vi "sinh fitter.vi"(3 "iterations":u16=1 min=1, 4 "1/B":dbl format="%.3f", 5 "amp.":dbl[](array[numeric]) format="%.2f", 6 "T":dbl[](array[numeric]) format="%.2f") -> (0 "sum of square deviations":dbl format="%.2f", 1 "a":dbl format="%.2f", 2 "m*":dbl format="%.2f")   [LabVIEW 2016]
uses:
  <vilib>/Analysis/baseanly.llb/Real Dot Product.vi
  <vilib>/Analysis/NI_AALBase.lvlib
  <vilib>/Analysis/NI_AALPro.lvlib
panel:
  out "plotted data":cluster{dbl[], dbl[]}[](graph)
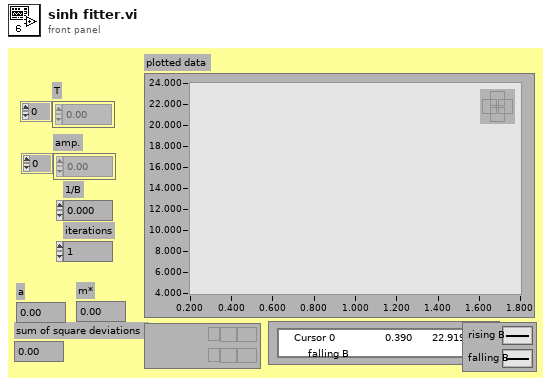
[diagram p1: front panel]
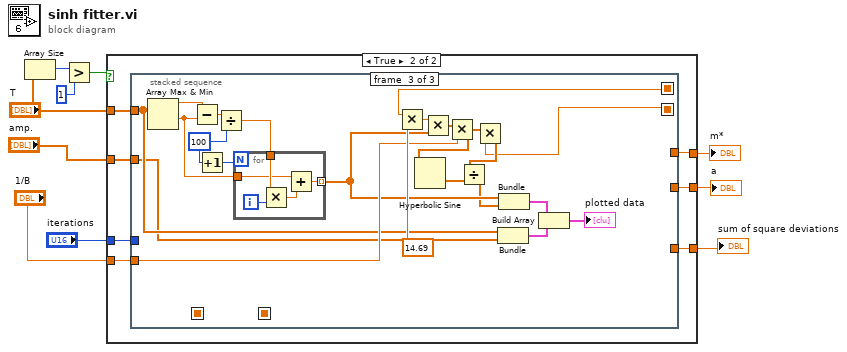
[diagram p0: block diagram]
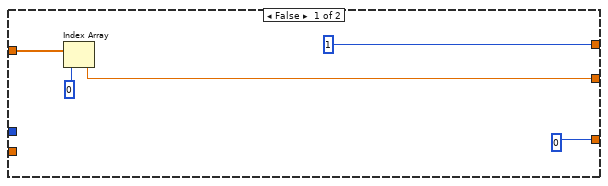
[diagram p2: hidden frame]
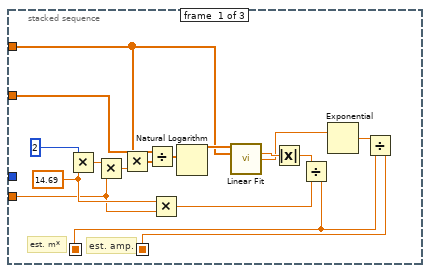
[diagram p3: hidden frame]
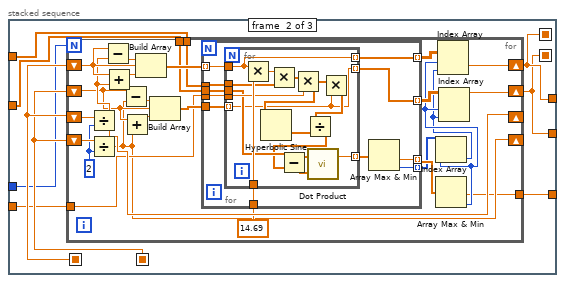
[diagram p4: hidden frame]
diagram:
  n1 = Array Size(array="T") -> (size(s)=w8:i32)
  n2 = Greater?(x=w8, y=1) -> (0:w7:bool)
  n3 = case shown="True" w7 {
    tunnel: [1 w19] -> w6
    tunnel: "T" -> [_ w22]
    tunnel: "amp." -> [w13 w21]
    tunnel: "1/B" -> [_ w20]
    tunnel: "iterations" -> [_ w18]
    tunnel: [w12 w17] -> w2
    tunnel: [0 w16] -> w1
    frame False {
      n4 = Index Array(array=w13, index=0) -> (element=w12:dbl)
    }
    frame True {
      n5 = stacked-sequence {
        seq-local: [w23 _ _] -> [_ w48 _]
        seq-local: [w24 _ _] -> [_ w47 _]
        seq-local: [_ w41 _] -> [_ _ w109]
        seq-local: [_ w40 _] -> [_ _ w107]
        tunnel: w22 -> [w32 w46 w104]
        tunnel: w21 -> [w35 w44 w103]
        tunnel: w20 -> [w30 w45 w108]
        tunnel: [_ w41 _] -> w19
        tunnel: w18 -> [_ w43 _]
        tunnel: [_ w40 _] -> w17
        tunnel: [_ w42 _] -> w16
        frame #0 {
          w31 = 14.69
          # "est. amp."
          # "est. m*"
          n6 = Multiply(x=2, y=w31) -> (x*y=w38:dbl)
          n7 = Multiply(x=w38, y=w30) -> (x*y=w37:dbl)
          n8 = Multiply(x=w32, y=w37) -> (x*y=w36:dbl[])
          n9 = Divide(x=w35, y=w36) -> (x/y=w34:dbl[])
          n10 = Multiply(x=w31, y=w30) -> (x*y=w28:dbl)
          n11 = Natural Logarithm(1:w34) -> (0:w33:dbl[])
          n12 = call <vilib>:"Linear Fit.vi"("Y"=w33, "X"=w32) -> ("slope"=w29:dbl, "intercept"=w26:dbl)  [unwired: 9 in, 3 out]
          n13 = Absolute Value(x=w29) -> (abs(x)=w27:dbl)
          n14 = Divide(x=w27, y=w28) -> (x/y=w23:dbl)
          n15 = Exponential(1:w26) -> (0:w25:dbl)
          n16 = Divide(x=w25, y=w23) -> (x/y=w24:dbl)
        }
        frame #1 {
          n17 = for {
            N: w43 -> [_]
            shift-right: [w71] -> _
            shift-left: w48 -> [w74]
            shift-right: [w53] -> _
            shift-left: w47 -> [w73]
            shift-right: [w55] -> w41
            shift-left: w48 -> [w72]
            shift-right: [w54] -> w40
            shift-left: w47 -> [w61]
            tunnel: w46 -> [w63]
            tunnel: w45 -> [w62]
            tunnel: w44 -> [w60]
            tunnel: [w49] -> w42
            w50 = 2
            n18 = Divide(x=w74, y=w50) -> (x/y=w71:dbl)
            n19 = Divide(x=w73, y=w50) -> (x/y=w53:dbl)
            n20 = Subtract(x=w72, y=w71) -> (x-y=w69:dbl)
            n21 = Add(x=w72, y=w71) -> (x+y=w70:dbl)
            n22 = Subtract(x=w61, y=w53) -> (x-y=w68:dbl)
            n23 = Add(x=w61, y=w53) -> (x+y=w67:dbl)
            n24 = Build Array(w69, w72, w70) -> (w66:dbl[])
            n25 = Build Array(w68, w61, w67) -> (w65:dbl[])
            n26 = for {
              tunnel: w66 -> [w85] mode=indexing
              tunnel: w65 -> [w84]
              tunnel: 14.69 -> [w83]
              tunnel: w63 -> [w82]
              tunnel: w62 -> [w81]
              tunnel: w60 -> [w80]
              tunnel: [w79] -> w57 mode=indexing
              tunnel: [w78] -> w56 mode=indexing
              tunnel: [w76] -> w59 mode=indexing
              tunnel: [w75] -> w58 mode=indexing
              n27 = for {
                tunnel: w85 -> [w87]
                tunnel: w84 -> [w86] mode=indexing
                tunnel: w83 -> [w99]
                tunnel: w82 -> [w97]
                tunnel: w81 -> [w95]
                tunnel: w80 -> [w91]
                tunnel: [w88] -> w77 mode=indexing
                tunnel: [w87] -> w79 mode=indexing
                tunnel: [w86] -> w78 mode=indexing
                n28 = Multiply(x=w87, y=w99) -> (x*y=w98:dbl)
                n29 = Multiply(x=w98, y=w97) -> (x*y=w96:dbl[])
                n30 = Multiply(x=w96, y=w95) -> (x*y=w94:dbl[])
                n31 = Hyperbolic Sine(1:w94) -> (0:w92:dbl[])
                n32 = Multiply(x=w94, y=w86) -> (x*y=w93:dbl[])
                n33 = Divide(x=w93, y=w92) -> (x/y=w90:dbl[])
                n34 = Subtract(x=w91, y=w90) -> (x-y=w89:dbl[])
                n35 = call-poly <vilib>:"Dot Product.vi"("Y Vector"=w89, "X Vector"=w89) -> ("X * Y"=w88:dbl)  [unwired: 1 out]
              }
              n36 = Array Max & Min(array=w77) -> (min value=w76:dbl, min index (indices)=w75:i32)  [unwired: 2 out]
            }
            n37 = Array Max & Min(array=w59) -> (min value=w49:dbl, min index (indices)=w52:i32)  [unwired: 2 out]
            n38 = Index Array(array=w58, index=w52) -> (element=w51:i32)
            n39 = Index Array(array=w57, index (row)=w52, index (col)=w51) -> (element=w55:dbl)
            n40 = Index Array(array=w56, index (row)=w52, index (col)=w51) -> (element=w54:dbl)
          }
        }
        frame #2 {
          w113 = 100
          n41 = Array Max & Min(array=w104) -> (max value=w115:dbl, min value=w110:dbl)  [unwired: 2 out]
          n42 = Subtract(x=w115, y=w110) -> (x-y=w114:dbl)
          n43 = Increment(x=w113) -> (x+1=w112:i32)
          n44 = Divide(x=w114, y=w113) -> (x/y=w111:dbl)
          n45 = for {
            N: w112 -> [_]
            tunnel: w111 -> [w126]
            tunnel: w110 -> [w123]
            tunnel: [w122] -> w106 mode=indexing
            i -> [w125]
            n46 = Multiply(x=w126, y=w125) -> (x*y=w124:dbl)
            n47 = Add(x=w123, y=w124) -> (x+y=w122:dbl)
          }
          n48 = Multiply(x=w109, y=14.69) -> (x*y=w121:dbl)
          n49 = Multiply(x=w121, y=w106) -> (x*y=w120:dbl[])
          n50 = Multiply(x=w120, y=w108) -> (x*y=w119:dbl[])
          n51 = Hyperbolic Sine(1:w119) -> (0:w117:dbl[])
          n52 = Multiply(x=w119, y=w107) -> (x*y=w118:dbl[])
          n53 = Divide(x=w118, y=w117) -> (x/y=w105:dbl[])
          n54 = Bundle("T"=w104, "amp."=w103) -> (w101:cluster{"T":dbl[], "amp.":dbl[]})  [unwired: 1 in]
          n55 = Bundle(w106, w105) -> (w102:cluster{dbl[], dbl[]})  [unwired: 1 in]
          n56 = Build Array(w102, w101) -> (→"plotted data":cluster{"T":dbl[], "amp.":dbl[]}[])
        }
      }
    }
  }
  "m*" <- w6
  "a" <- w2
  "sum of square deviations" <- w1
